vi "test_fast_PID_chain.vi"() -> ()   [LabVIEW 2013]
uses:
  <vilib>/measure/NI_MABase.lvlib
  Scope5782/Scope/controls/Memory block.ctl
panel:
  out "Waveform Graph 4":dbl[](graph)
  out "Waveform Graph 3":dbl[][](graph)
  out "Waveform Graph 2":i16[](graph)
  out "Waveform Graph":dbl[](graph)
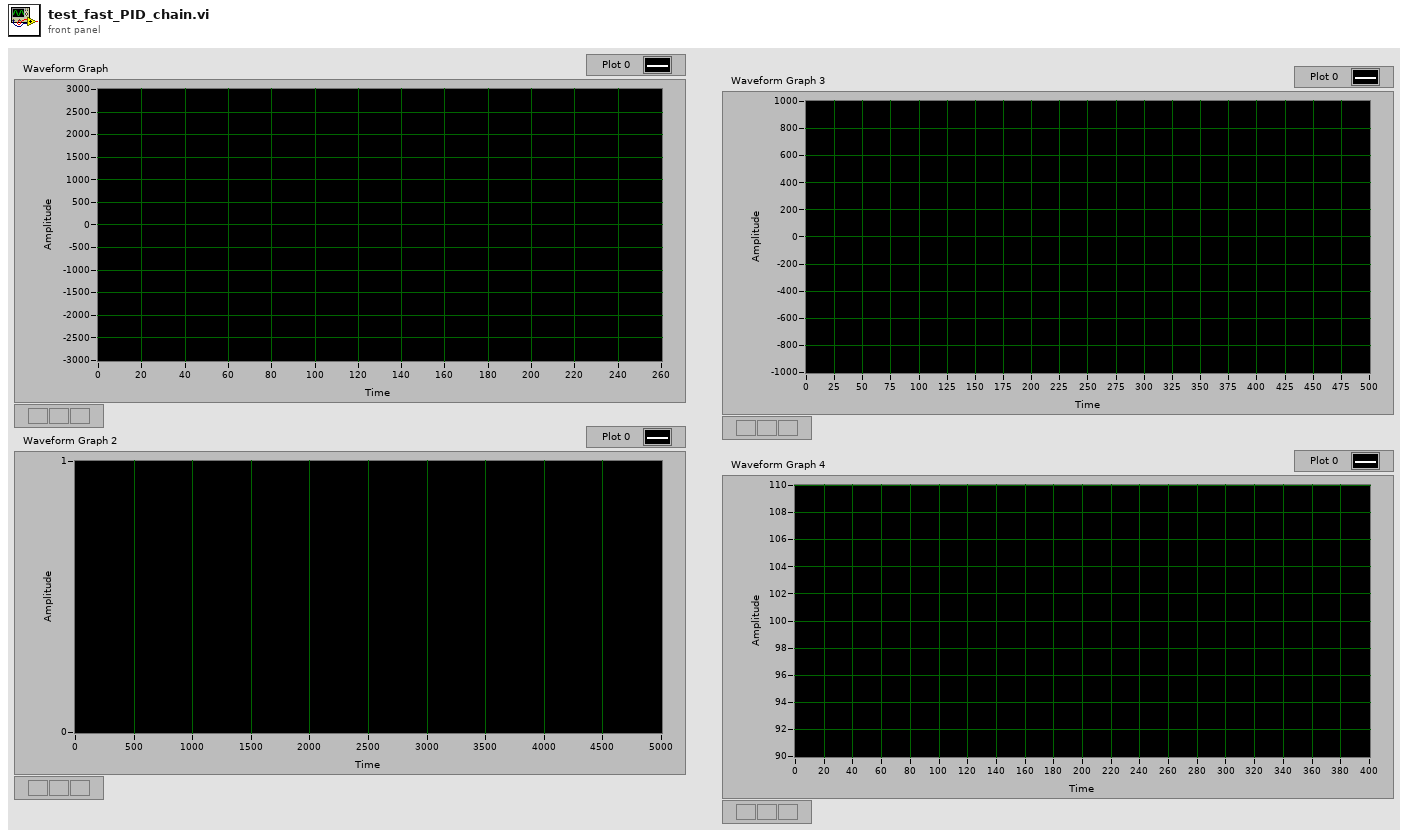
[diagram p1: front panel]
types:
  T1 = typedef "Memory block.ctl" = enum16{"Setpoint", "Beam"}
  T2 = cluster{"frequency":dbl, "amplitude":dbl, "phase":dbl}[]
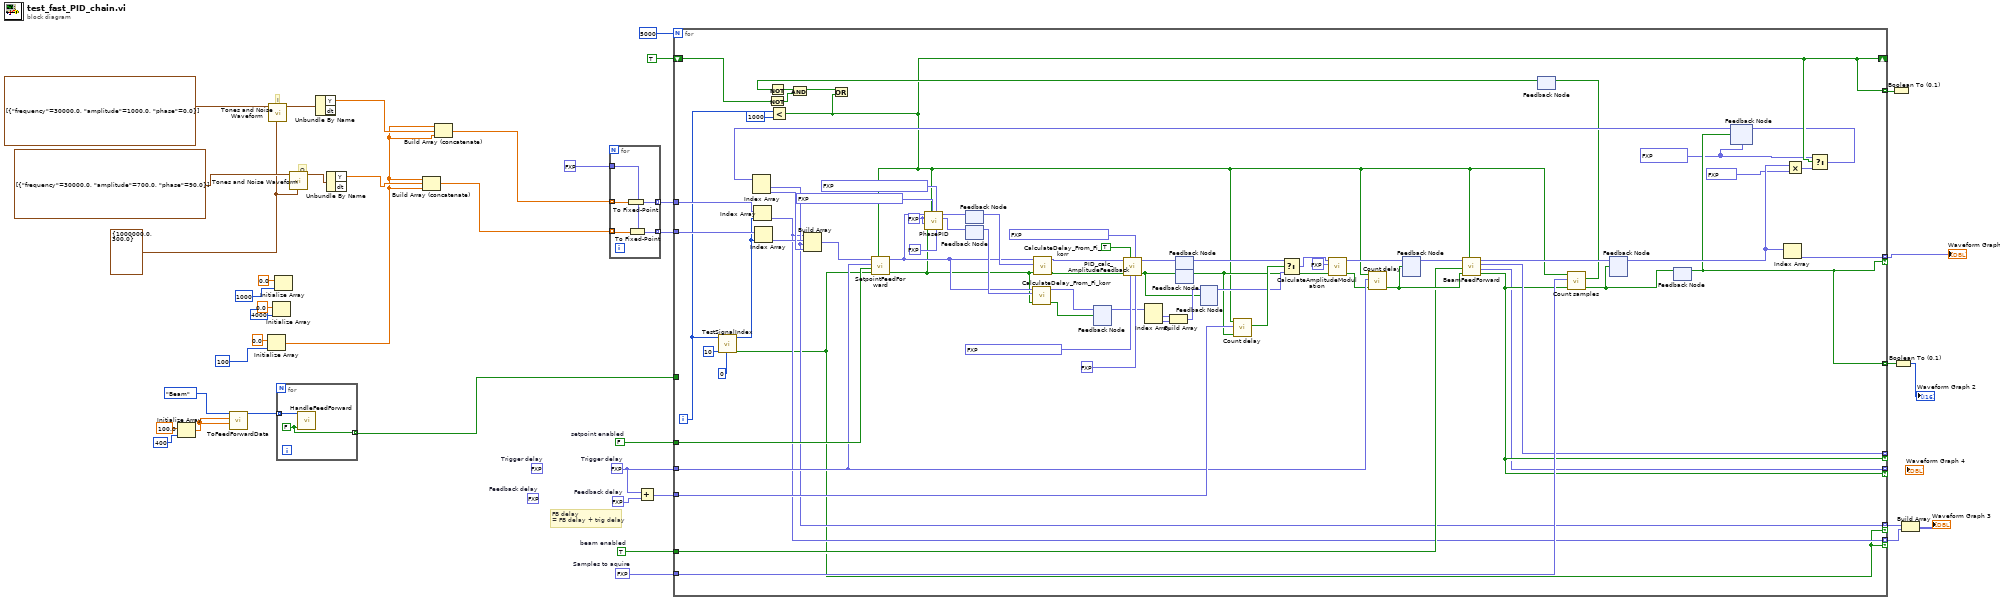
[diagram p0: block diagram]
diagram:
  (unwired) fxp<+/-,16,16> 10.0  # Feedback delay
  (unwired) fxp<+/-,16,16> 25.0  # Trigger delay
  w28 = TRUE  # beam enabled
  w29 = fxp<+,16,16> 250.0  # Samples to aquire
  w30 = FALSE  # setpoint enabled
  w33 = fxp<+/-,16,16> 0.0  # Feedback delay
  w31 = fxp<+/-,16,16> 0.0  # Trigger delay
  w26 = cluster{"Fs":dbl, "#s":dbl} {"Fs"=1000000.0, "#s"=300.0} ("sampling info")
  # "Q"
  # "I"
  # "FB delay\n= FB delay + trig delay"
  n1 = Initialize Array(100.0 ("element"), 400 ("dimension size")) -> (w4:dbl[])
  n2 = call "ToFeedForwardData.vi"("values Q"=w4, "values I"=w4, "Memory block"=Memory_block."Beam") -> ("Data"=w8:u64[])  [unwired: 8 in]
  n3 = Initialize Array(0.0 ("element"), 100 ("dimension size")) -> (w16:dbl[])
  n4 = call <vilib>:"Tones and Noise Waveform.vi"("sampling info"=w26, "tones"=T2 [{"frequency"=30000.0, "amplitude"=1000.0, "phase"=0.0}]) -> ("signal out"=w38:waveform(dbl))  [unwired: 8 in, 1 out]
  n5 = Initialize Array(0.0 ("element"), 4000 ("dimension size")) -> ()  [unwired: 1 out]
  n6 = Initialize Array(0.0 ("element"), 1000 ("dimension size")) -> ()  [unwired: 1 out]
  n7 = for {
    tunnel: w8 -> [w42] mode=indexing
    tunnel: [w41] -> w1 mode=indexing
    w41 = FALSE ("timed out")
    n8 = call "HandleFeedForward.vi"("timed out"=w41, "Value"=w42) -> ()  [unwired: 8 in, 2 out]
  }
  n9 = call <vilib>:"Tones and Noise Waveform.vi"("sampling info"=w26, "tones"=T2 [{"frequency"=30000.0, "amplitude"=700.0, "phase"=90.0}]) -> ("signal out"=w23:waveform(dbl))  [unwired: 8 in, 1 out]
  n10 = Unbundle By Name(w38) -> ("Y"=w19:dbl[])  [unwired: 1 out]
  n11 = Unbundle By Name(w23) -> ("Y"=w18:dbl[])  [unwired: 1 out]
  n12 = Build Array (concatenate)(w16, w18, w16) -> (w15:dbl[])
  n13 = Build Array (concatenate)(w16, w19, w16) -> (w10:dbl[])
  n14 = for {
    tunnel: w15 -> [w46] mode=indexing
    tunnel: fxp<+/-,16,14> 0.0 ("fixed-point type") -> [w47]
    tunnel: [w45] -> w37 mode=indexing
    tunnel: w10 -> [w43] mode=indexing
    tunnel: [w44] -> w14 mode=indexing
    n15 = To Fixed-Point(number=w43) -> (fixed-point=w44:fxp<+/-,16,14>)  [unwired: 1 in]
    n16 = To Fixed-Point(fixed-point type=w47, number=w46) -> (fixed-point=w45:fxp<+/-,16,14>)
  }
  n17 = Add(x=w31, y=w33) -> (x+y=w32:fxp<+/-,17,17>)
  n18 = for {
    N: 5000 -> [_]
    tunnel: w37 -> [w117]
    tunnel: [w79] -> w36 mode=indexing
    tunnel: [w116] -> w34 mode=indexing if=w79
    tunnel: w32 -> [w115]
    tunnel: w31 -> [w86]
    tunnel: w30 -> [w114]
    tunnel: w29 -> [w88]
    tunnel: w28 -> [w87]
    tunnel: w14 -> [w85]
    shift-right: [w59] -> _
    shift-left: TRUE -> [w74]
    tunnel: [w59] -> w11 mode=indexing
    tunnel: [w51] -> _ mode=indexing if=w52
    tunnel: [w53] -> _ mode=indexing if=w52
    tunnel: [w50] -> w3 mode=indexing if=w48
    tunnel: [w49] -> w2 mode=indexing if=w48
    tunnel: w1 -> [_]
    i -> [w78]
    w57 = fxp<+/-,21,13>[] [0.0, 0.0]
    w65 = fxp<+/-,32,4> 0.0 ("Fi_start")
    n19 = call "TestSignalIndex.vi"("initial delay"=0, "cycles per sample"=10, "index"=w78) -> ("valid out"=w48:bool, "array index"=w69:i32)  [unwired: 7 in]
    n20 = Index Array(array=w85, index=w69) -> (element=w49:fxp<+/-,16,14>)
    n21 = Index Array(array=w117, index=w69) -> (element=w70:fxp<+/-,16,14>)
    n22 = Not(x=w74) -> (.not. x?=w72:bool)
    n23 = Less?(x=w78, y=1000) -> (x < y?=w59:bool)
    n24 = feedback #1() -> (w63:fxp<+/-,32,4>)  [unwired: 1 in]
    n25 = feedback #2() -> (w61:fxp<+/-,32,4>)  [unwired: 1 in]
    n26 = feedback #3() -> (w95:fxp<+/-,16,14>[])  [unwired: 1 in]
    n27 = Index Array(array=w95) -> (element #1=w97:fxp<+/-,16,14>, element #2=w96:fxp<+/-,16,14>)  [unwired: 2 in]
    n28 = Build Array(w97, w96) -> (w94:fxp<+/-,16,14>[])
    n29 = feedback #4() -> (w99:fxp<+/-,16,14>[])  [unwired: 1 in]
    n30 = feedback #5() -> (w102:bool)  [unwired: 1 in]
    n31 = feedback #6() -> (w103:fxp<+/-,16,14>[])  [unwired: 1 in]
    n32 = call "Count delay.vi"("input valid"=w102, "Count to skip"=w115, "Reset"=w59) -> ("count done?"=w104:bool)  [unwired: 7 in, 1 out]
    n33 = Select(t=w99, s=w104, f=w103) -> (s? t:f=w98:fxp<+/-,16,14>[])
    n34 = call "CalculateAmplitudeModulation.vi"("input valid"=w102, "AM_factor"=fxp<+/-,16,2> 1.0, "Data in"=w98) -> ("output valid"=w80:bool, "Data out"=w112:fxp<+/-,16,14>[])  [unwired: 7 in]
    n35 = call "Count delay.vi"("input valid"=w80, "Count to skip"=w86, "Reset"=w59) -> ("output valid"=w91:bool)  [unwired: 7 in, 1 out]
    n36 = feedback #7() -> (w93:fxp<+/-,16,14>[])  [unwired: 1 in]
    n37 = feedback-in #7(w112, w91) -> ()
    n38 = call "BeamFeedForward.vi"("Reset"=w59, "input valid"=w91, "beam enabled"=w87, "Data in"=w93) -> ("output valid"=w52:bool, "Data"=w51:fxp<+/-,16,14>, "Data 2"=w53:fxp<+/-,16,14>, "Data out"=w92:fxp<+/-,16,14>[])  [unwired: 4 in]
    n39 = feedback #8() -> (w75:bool)  [unwired: 1 in]
    n40 = Not(x=w75) -> (.not. x?=w73:bool)
    n41 = And(x=w73, y=w72) -> (x .and. y?=w71:bool)
    n42 = Or(x=w71, y=w59) -> ()  [unwired: 1 out]
    n43 = call "Count samples.vi"("input valid"=w52, "Samples to count"=w88, "Reset"=w59) -> ("output valid"=w105:bool, "counting"=w76:bool)  [unwired: 7 in]
    n44 = feedback-in #8(w76) -> ()
    n45 = feedback #9() -> (w84:fxp<+/-,16,14>[])  [unwired: 1 in]
    n46 = feedback-in #9(w92, w105) -> ()
    n47 = feedback #10() -> (w79:bool)  [unwired: 1 in]
    n48 = feedback-in #10(w105) -> ()
    n49 = feedback #11(w57) -> (w82:fxp<+/-,21,13>[])
    n50 = Index Array(array=w82) -> (element #1=w50:fxp<+/-,21,13>, element #2=w81:fxp<+/-,21,13>)  [unwired: 2 in]
    n51 = Build Array(w49, w70, w50, w81) -> (w56:fxp<+/-,22,14>[])
    n52 = call "SetpointFeedForward.vi"("Reset"=w59, "input valid"=w48, "setpoint enabled"=w114, "Samples to skip"=w86, "Data in"=w56) -> ("output valid"=w54:bool, "Data out"=w55:fxp<+/-,16,14>[])  [unwired: 5 in]
    n53 = call "PhasePID.vi"("Kd/Tau"=fxp<+/-,32,4> 0.0, "Ki*Tau"=fxp<+/-,32,4> 0.000999998301267624, "Kp"=fxp<+/-,32,4> 0.010000001639127731, "Reset"=w59, "input valid"=w54, "Fi_delta"=w65, "Fi_start"=w65, "Data in"=w55) -> ("Fi_korr"=w62:fxp<+/-,32,4>, "Fi_korr PID"=w64:fxp<+/-,32,4>)  [unwired: 1 in, 1 out]
    n54 = feedback-in #1(w64) -> ()
    n55 = feedback-in #2(w62) -> ()
    n56 = call "CalculateDelay_From_Fi_korr.vi"("input valid"=w54, "fi_korr"=w61, "Data in"=w55) -> ("output valid"=w100:bool, "Data out"=w101:fxp<+/-,16,14>[])  [unwired: 7 in]
    n57 = call "CalculateDelay_From_Fi_korr.vi"("input valid"=w54, "fi_korr"=w63, "Data in"=w55) -> ("output valid"=w107:bool, "Data out"=w106:fxp<+/-,16,14>[])  [unwired: 7 in]
    n58 = feedback-in #3(w101, w100) -> ()
    n59 = call "PID_calc_AmplitudeFeedback.vi"("Kd/Tau"=fxp<+/-,32,6> 0.0 ("Data"), "Ki*Tau"=fxp<+/-,32,6> 0.0010000020265579224 ("Data"), "Kp"=fxp<+/-,32,6> 0.010000020265579224 ("Data"), "Enabled"=TRUE, "input valid"=w107, "Data in"=w106) -> ("output valid"=w89:bool, "data out"=w90:fxp<+/-,16,14>[])  [unwired: 2 in, 2 out]
    n60 = feedback-in #4(w90) -> ()
    n61 = feedback-in #5(w89) -> ()
    n62 = feedback-in #6(w94, w89) -> ()
    n63 = Index Array(array=w84) -> (element=w116:fxp<+/-,16,14>)  [unwired: 1 in]
    n64 = Multiply(x=w84, y=fxp<+,5,-1> 0.296875 ("Q out")) -> (x*y=w60:fxp<+/-,21,13>[])
    n65 = Select(t=w57, s=w59, f=w60) -> (s? t:f=w58:fxp<+/-,21,13>[])
    n66 = feedback-in #11(w58, w79) -> ()
  }
  "Waveform Graph" <- w34
  n67 = Boolean To (0,1)(Boolean=w11) -> ()  [unwired: 1 out]
  n68 = Boolean To (0,1)(Boolean=w36) -> (0, 1=→"Waveform Graph 2":i16[])
  n69 = Build Array(w3, w2) -> (→"Waveform Graph 3":fxp<+/-,22,14>[][])
